vi "Full close MV.vi"(8 "error in (no error)":errorcluster, 11 "Stand in":refnum<class "Stand.lvclass">) -> (0 "error out":errorcluster)   [LabVIEW 2019, in "Stand.lvclass"]
uses:
  Stand.lvclass
  Stand.lvclass/Stand.ctl
  Device_class/Device.lvclass/Device.ctl
  NeedleValve_class/NeedleValve.lvclass
  C:/Users/ANENKOV_V1/Desktop/src/Device_class/Device.lvclass
  MessageInterface_class/MessageInterface.lvclass
  Device_class/Device.lvclass
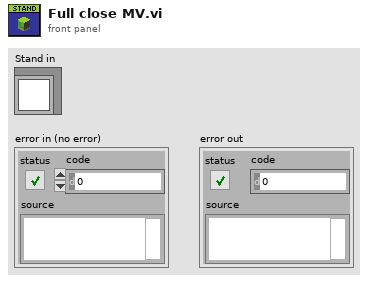
[diagram p1: front panel]
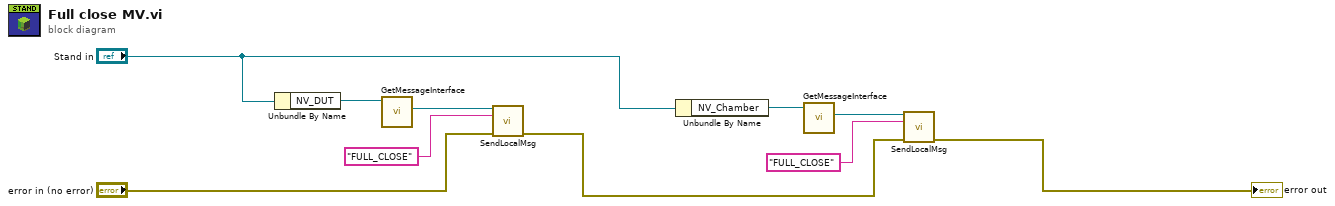
[diagram p0: block diagram]
diagram:
  n1 = Unbundle By Name("Stand in") -> ("NV_DUT"=w8:refnum<class "NeedleValve.lvclass">)
  n2 = call "GetMessageInterface.vi"("Device in"=w8) -> ("MessageInterface"=w4:refnum<class "MessageInterface.lvclass">)  [unwired: 10 in]
  n3 = call-dynamic "SendLocalMsg.vi"("reference in"=w4, "name"="FULL_CLOSE", "error in (no error)"="error in (no error)") -> ("error out"=w10:errorcluster)  [unwired: 10 in, 2 out]
  n4 = Unbundle By Name("Stand in") -> ("NV_Chamber"=w9:refnum<class "NeedleValve.lvclass">)
  n5 = call "GetMessageInterface.vi"("Device in"=w9) -> ("MessageInterface"=w7:refnum<class "MessageInterface.lvclass">)  [unwired: 10 in]
  n6 = call-dynamic "SendLocalMsg.vi"("reference in"=w7, "name"="FULL_CLOSE", "error in (no error)"=w10) -> ("error out"=→"error out":errorcluster)  [unwired: 10 in, 2 out]
